vi "即時計算式.vi"(0 "b y":i32, 5 "OK Button":bool, 7 "Va":dbl, 9 "Vc":dbl, 11 "S0":i32, 12 "H":dbl, 13 "stop":bool, 14 "ti":dbl) -> (2 "Disabled":T1(ring), 4 "b y 2":dbl, 6 "output stop":bool, 8 "a x":dbl, 10 "c x":dbl, 15 "to":dbl)   [LabVIEW 2014]
panel:
  out "k":dbl
  out "投彈時間(k)":dbl
  in  "S0":i32=630
  in  "Vc":dbl=30.0
  in  "Va":dbl=120.0
  in  "H":dbl=122.5
  in  "stop":bool
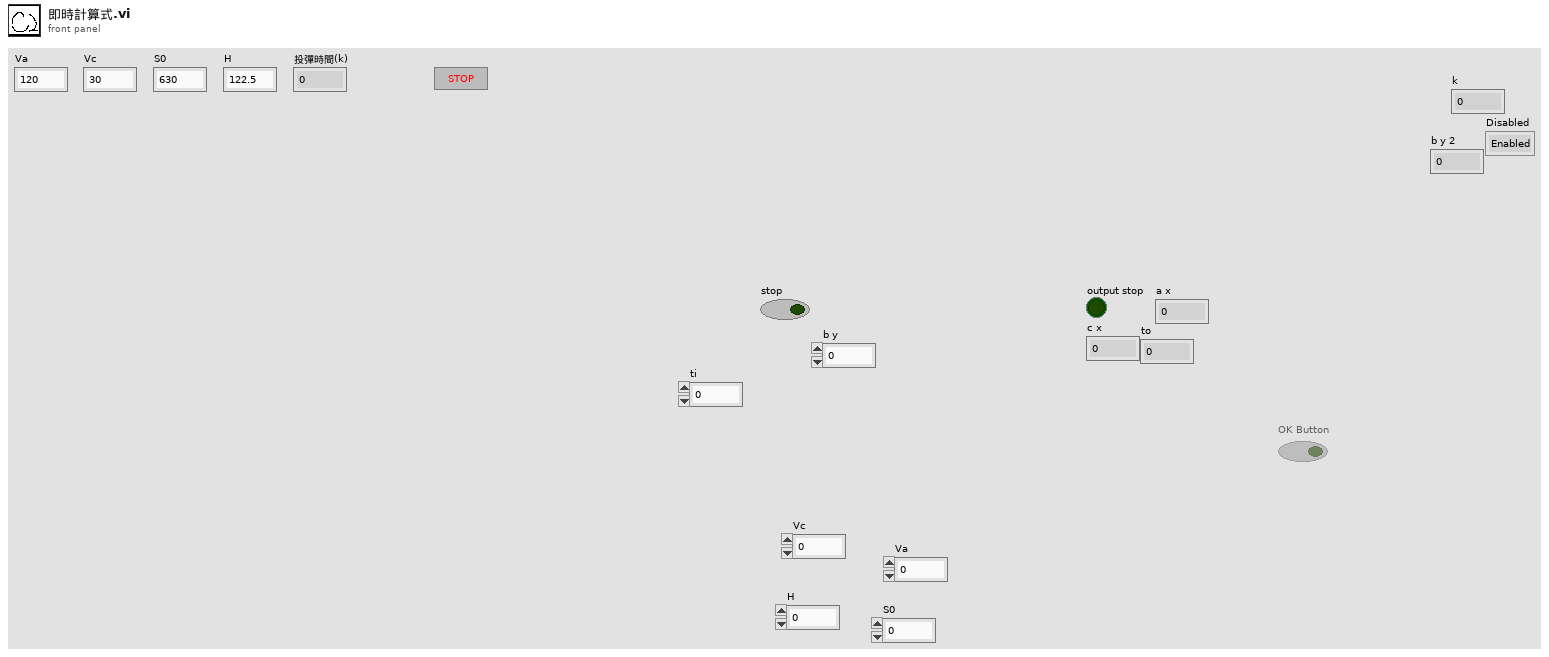
[diagram p1: front panel]
types:
  T1 = enum8{"Enabled", "Disabled", "Disabled and Grayed Out"}
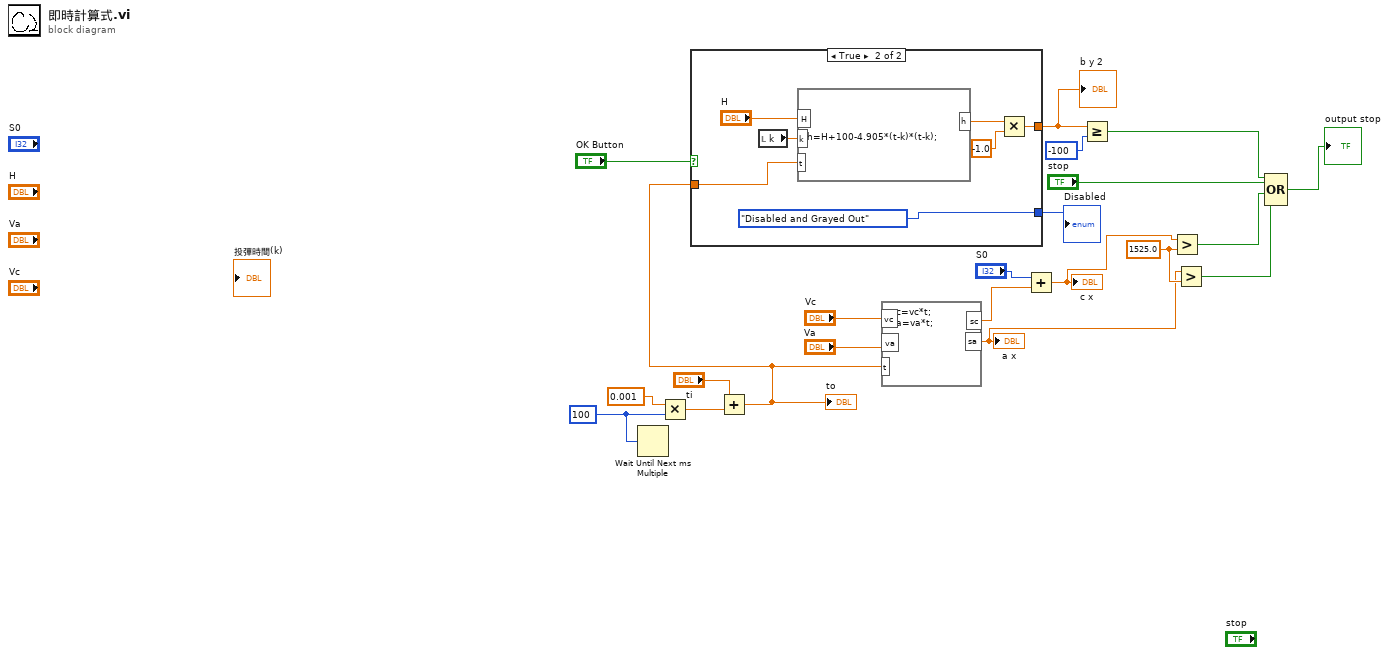
[diagram p0: block diagram]
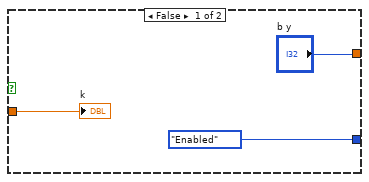
[diagram p2: hidden frame]
diagram:
  w6 = 1525.0 ("y")
  w21 = u32 100
  n1 = Wait Until Next ms Multiple(millisecond multiple=w21) -> ()  [unwired: 1 out]
  n2 = Multiply(x=0.001, y=w21) -> (x*y=w20:dbl)
  n3 = Add(x="ti", y=w20) -> (x+y=w15:dbl)
  "to" <- w15
  n4 = case shown="True" "OK Button" {
    tunnel: ["b y" w30] -> w18
    tunnel: w15 -> [w23 w29]
    tunnel: [T1."Enabled" ("Disabled") T1."Disabled and Grayed Out" ("Disabled")] -> w9
    frame False {
      "k" <- w23
    }
    frame True {
      n5 = local read "k"() -> (w26:dbl)
      n6 = formula code="h=H+100-4.905*(t-k)*(t-k);"("H"="H", "t"=w29, "k"=w26) -> ("h"=w31:dbl)
      n7 = Multiply(x=w31, y=-1.0) -> (x*y=w30:dbl)
    }
  }
  "b y 2" <- w18
  "Disabled" <- w9
  n8 = formula code="sc=vc*t;\nsa=va*t;"("vc"="Vc", "t"=w15, "va"="Va") -> ("sc"=w16:dbl, "sa"=w4:dbl)
  "a x" <- w4
  n9 = Add(x="S0", y=w16) -> (x+y=w5:dbl)
  "c x" <- w5
  n10 = Greater Or Equal?(x=w18, y=-100) -> (x >= y?=w8:bool)
  n11 = Greater?(x=w5, y=w6) -> (0:w3:bool)
  n12 = Greater?(x=w4, y=w6) -> (0:w2:bool)
  n13 = Compound Arithmetic op=OR(w8, "stop", w3, w2) -> (→"output stop":bool)
